vi "Check If Unique lvlib.vi"(9 "Type Name Library File Path":map{string, map{string, path}}(c390), 10 "Library File Path":path) -> (2 "Unique?":bool)   [LabVIEW 2020, in "_Shared.lvlib"]
uses:
  _Shared.lvlib
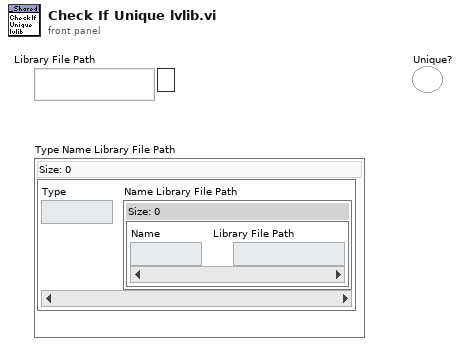
[diagram p1: front panel]
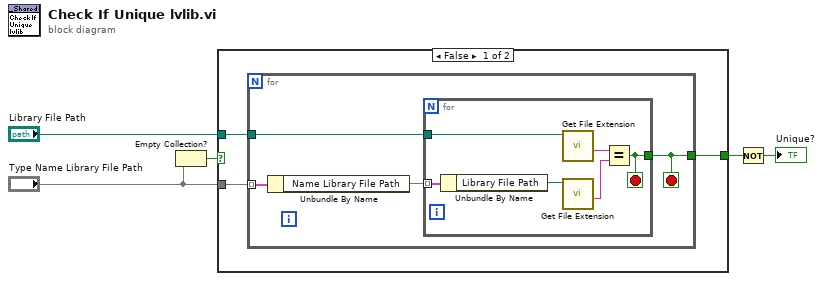
[diagram p0: block diagram]
diagram:
  n1 = Empty Collection?(1:"Type Name Library File Path") -> (0:w5:bool)
  n2 = case shown="False" w5 {
    tunnel: "Library File Path" -> [w8 _]
    tunnel: [w6 _] -> w2
    tunnel: "Type Name Library File Path" -> [w7 _]
    frame False {
      n3 = for {
        tunnel: w7 -> [w12] mode=indexing
        tunnel: w8 -> [w10]
        tunnel: [w9] -> w6
        stop <- w9 stop-if-true
        n4 = Unbundle By Name(w12) -> ("Name Library File Path"=w11:map{string, path})
        n5 = for {
          tunnel: w11 -> [w18] mode=indexing
          tunnel: w10 -> [w16]
          tunnel: [w17] -> w9
          stop <- w17 stop-if-true
          n6 = Unbundle By Name(w18) -> ("Library File Path"=w14:path)
          n7 = call <vilib>:"Get File Extension.vi"("file"=w16) -> ("filename without extension"=w15:string)  [unwired: 6 in, 4 out]
          n8 = call <vilib>:"Get File Extension.vi"("file"=w14) -> ("filename without extension"=w13:string)  [unwired: 6 in, 4 out]
          n9 = Equal?(x=w15, y=w13) -> (x = y?=w17:bool)
        }
      }
    }
    frame True {
    }
  }
  n10 = Not(x=w2) -> (.not. x?=→"Unique?":bool)
